vi "expanded_index_array.vi"(10 "start":i32, 11 "values":dbl[](array[numeric])) -> (1 "third":dbl, 2 "second":dbl, 3 "first":dbl)   [LabVIEW 2020]
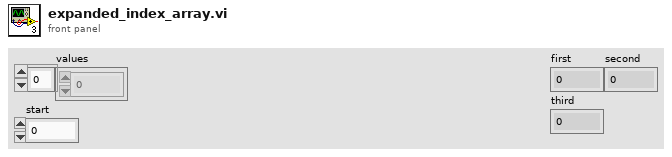
[diagram p1: front panel]
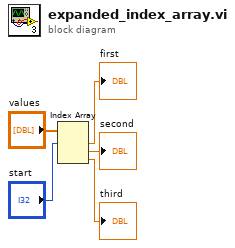
[diagram p0: block diagram]
diagram:
  n1 = Index Array(array="values", index #1="start") -> (element #1=→"first":dbl, element #2=→"second":dbl, element #3=→"third":dbl)  [unwired: 2 in]
